vi "Extended User Data.vi"(7 "Action":u16(ring) items=["Read Data", "Write Data", "Clear Data", "Clear ALL Data"], 8 "error in (no error)":errorcluster, 10 "User Data In":T1, 11 "VISA resource name":refnum<visa-resource-name>) -> (0 "error out":errorcluster, 2 "User Data Out":T1, 3 "VISA resource name out":refnum<visa-resource-name>)   [LabVIEW 2012, in "Agilent PSG MXG Series.lvlib"]
doc: "Writes, reads, and clears data of the type User Data In to the connected VISA session."
uses:
  <instrlib>/Agilent PSG MXG Series/Agilent PSG MXG Series.lvlib
  <instrlib>/Agilent PSG MXG Series/Private/Extended User Data.ctl
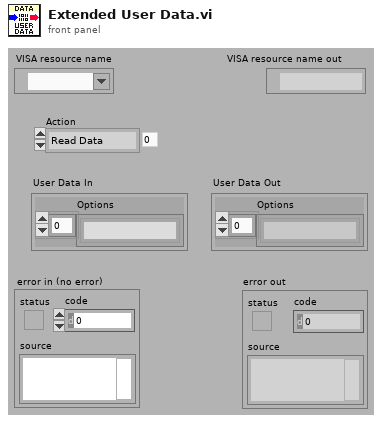
[diagram p1: front panel]
types:
  T1 = typedef "Agilent PSG MXG Series.lvlib/Extended User Data.ctl" = cluster{"Options":string[]}
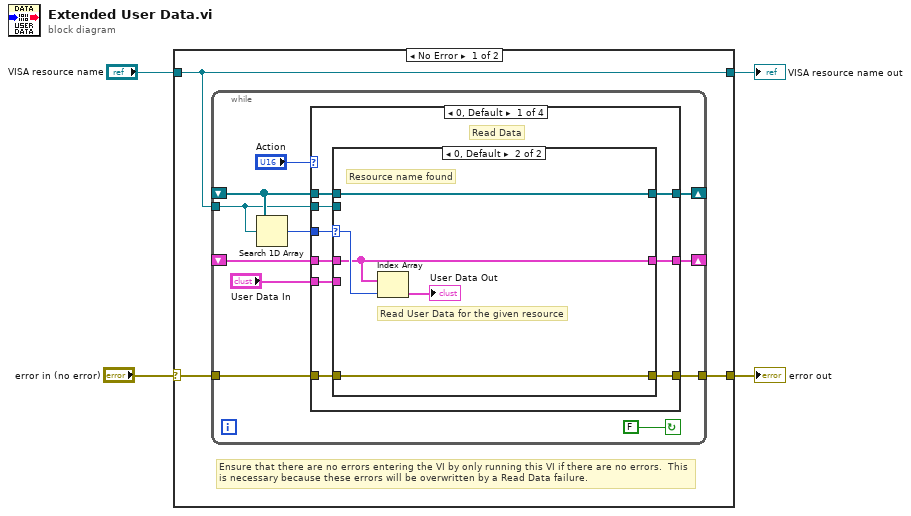
[diagram p0: block diagram]
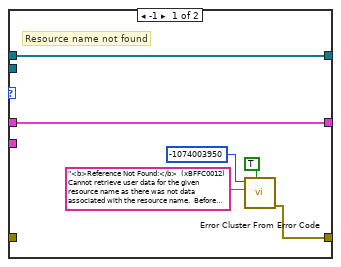
[diagram p2: hidden frame]
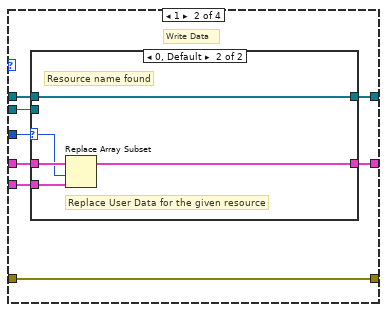
[diagram p3: hidden frame]
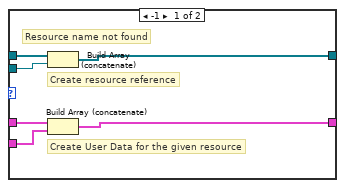
[diagram p4: hidden frame]
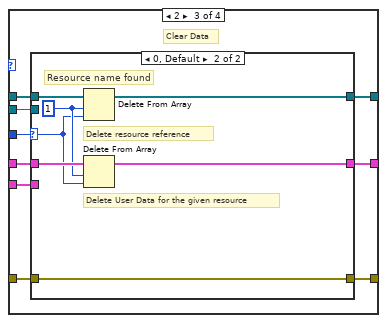
[diagram p5: hidden frame]
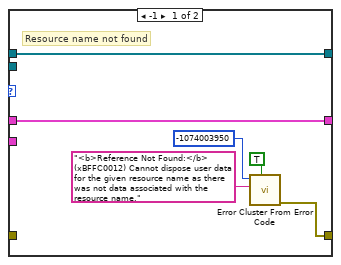
[diagram p6: hidden frame]
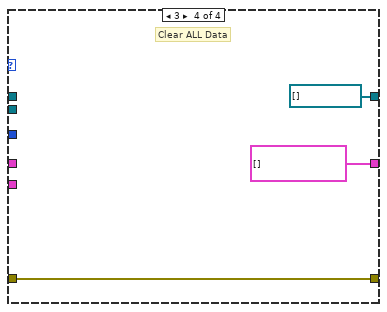
[diagram p7: hidden frame]
diagram:
  n1 = case shown="No Error" "error in (no error)" {
    selector: "error in (no error)" -> [w6 w84]
    tunnel: "VISA resource name" -> [w5 w83]
    tunnel: [w7 w84] -> w3
    tunnel: [w5 w83] -> w1
    frame No Error {
      # "Ensure that there are no errors entering the VI by only running this VI if there are no errors.  This is necessary because these errors will be overwritten by a Read Data failure."
      n2 = while {
        shift-right: [w14] -> _
        shift-left: _ -> [w15]
        shift-right: [w17] -> _
        shift-left: _ -> [w18]
        tunnel: w5 -> [w13]
        tunnel: w6 -> [w10]
        tunnel: [w9] -> w7
        stop <- FALSE continue-if-true
        n3 = Search 1D Array(1D array=w15, element=w13) -> (index of element=w16:i32)  [unwired: 1 out]
        n4 = case shown="0, Default" "Action" {
          tunnel: "User Data In" -> [w27 w46 w66 _]
          tunnel: w18 -> [w26 w45 w65 _]
          tunnel: [w25 w44 w64 T1[] []] -> w17
          tunnel: w16 -> [w24 w43 w63 _]
          tunnel: w15 -> [w23 w42 w62 _]
          tunnel: [w22 w41 w61 refnum<visa-resource-name>[] []] -> w14
          tunnel: w13 -> [w21 w40 w60 _]
          tunnel: w10 -> [w19 w39 w58 w80]
          tunnel: [w20 w39 w59 w80] -> w9
          frame 0, Default {
            # "Read Data"
            n5 = case shown="0, Default" w24 {
              selector: w24 -> [_ w38]
              tunnel: w27 -> [_ _]
              tunnel: [w32 w35] -> w25
              tunnel: w26 -> [w32 w35]
              tunnel: w23 -> [w33 w37]
              tunnel: [w33 w37] -> w22
              tunnel: w21 -> [_ _]
              tunnel: [w31 w34] -> w20
              tunnel: w19 -> [_ w34]
              frame -1 {
                # "Resource name not found"
                n6 = call <vilib>:"Error Cluster From Error Code.vi"("show call chain? (False)"=TRUE, "error message (\"\")"="<b>Reference Not Found:</b>  (xBFFC0012) Cannot retrieve user data for the given resource name as there was not data associated with the resource name.  Before you can read data, you need to write the user data using the Write Data action of this User Data VI. ", "error code (0)"=-1074003950 ("Code")) -> ("error out"=w31:errorcluster)  [unwired: 1 in, 5 out]
              }
              frame 0, Default {
                # "Read User Data for the given resource"
                # "Resource name found"
                n7 = Index Array(array=w35, index=w38) -> (element=→"User Data Out":T1)
              }
            }
          }
          frame 1 {
            # "Write Data"
            n8 = case shown="0, Default" w43 {
              selector: w43 -> [_ w54]
              tunnel: w46 -> [w50 w55]
              tunnel: [w49 w57] -> w44
              tunnel: w45 -> [w51 w56]
              tunnel: w42 -> [w52 w53]
              tunnel: [w47 w53] -> w41
              tunnel: w40 -> [w48 _]
              frame -1 {
                # "Create resource reference"
                # "Create User Data for the given resource"
                # "Resource name not found"
                n9 = Build Array (concatenate)(w52, w48) -> (w47:refnum<visa-resource-name>[])
                n10 = Build Array (concatenate)(w51, w50) -> (w49:T1[])
              }
              frame 0, Default {
                # "Replace User Data for the given resource"
                # "Resource name found"
                n11 = Replace Array Subset(array=w56, new element=w55, index=w54) -> (w57:T1[])
              }
            }
          }
          frame 2 {
            # "Clear Data"
            n12 = case shown="0, Default" w63 {
              selector: w63 -> [_ w73]
              tunnel: w66 -> [_ _]
              tunnel: [w71 w79] -> w64
              tunnel: w65 -> [w71 w78]
              tunnel: w62 -> [w72 w76]
              tunnel: [w72 w75] -> w61
              tunnel: w60 -> [_ _]
              tunnel: [w70 w77] -> w59
              tunnel: w58 -> [_ w77]
              frame -1 {
                # "Resource name not found"
                n13 = call <vilib>:"Error Cluster From Error Code.vi"("show call chain? (False)"=TRUE, "error message (\"\")"="<b>Reference Not Found:</b>  (xBFFC0012) Cannot dispose user data for the given resource name as there was not data associated with the resource name.", "error code (0)"=-1074003950 ("Code")) -> ("error out"=w70:errorcluster)  [unwired: 1 in, 5 out]
              }
              frame 0, Default {
                w74 = 1 ("length")
                # "Delete resource reference"
                # "Delete User Data for the given resource"
                # "Resource name found"
                n14 = Delete From Array(array=w76, length=w74, index=w73) -> (array with subset deleted=w75:refnum<visa-resource-name>[])  [unwired: 1 out]
                n15 = Delete From Array(array=w78, length=w74, index=w73) -> (array with subset deleted=w79:T1[])  [unwired: 1 out]
              }
            }
          }
          frame 3 {
            # "Clear ALL Data"
          }
        }
      }
    }
    frame Error {
    }
  }
  "error out" <- w3
  "VISA resource name out" <- w1
